vi "XYStage.GetProtectedEventsRegistration.vi"(8 "error in (no error)":errorcluster, 11 "XYStage in":refnum<class "XYStage.lvclass">) -> (0 "error out":errorcluster, 2 "XYStage Protected Events":refnum<event-registration>, 3 "XYStage out":refnum<class "XYStage.lvclass">)   [LabVIEW 2017, in "XYStage.lvclass"]
uses:
  XYStage.lvclass
  Typedefs/ProtectedEvents--Cluster.ctl
  Typedefs/ProtectedEvents--XYStage.StatusUpdated.ctl
  Typedefs/XYStage.Axis--Enum.ctl
  Typedefs/XYStage.DeviceStatus--Enum.ctl
  Typedefs/ProtectedEvents--XYStage.MoveResultReported.ctl
  Typedefs/Coordinates--Cluster.ctl
  Typedefs/Coordinates.Units--Cluster.ctl
  Typedefs/Coordinates.Counts--Cluster.ctl
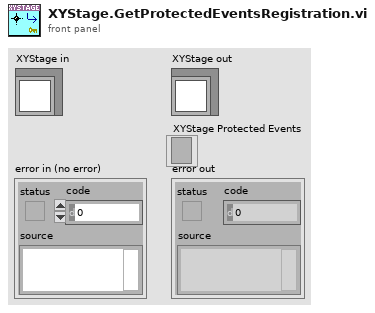
[diagram p1: front panel]
types:
  T1 = typedef "XYStage.lvclass/ProtectedEvents--Cluster.ctl" = cluster{"StatusUpdated":refnum<user-event>, "MoveResultReported":refnum<user-event>}
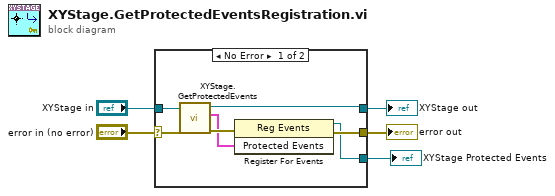
[diagram p0: block diagram]
diagram:
  n1 = case shown="No Error" "error in (no error)" {
    selector: "error in (no error)" -> [w9 w14]
    tunnel: [w12 w14] -> w4
    tunnel: [w7 w13] -> w2
    tunnel: "XYStage in" -> [w10 w13]
    tunnel: [w11 _] -> w1
    frame No Error {
      n2 = call "XYStage.GetProtectedEvents.vi"("error in (no error)"=w9, "XYStage"=w10) -> ("error out"=w8:errorcluster, "Protected Events"=w6:T1, "XYStage out"=w7:refnum<class "XYStage.lvclass">)  [unwired: 7 in]
      n3 = register-events(error in=w8, w6) -> (reference out=w11:refnum<event-registration>, error out=w12:errorcluster)  [unwired: 1 in]
    }
    frame Error {
    }
  }
  "error out" <- w4
  "XYStage out" <- w2
  "XYStage Protected Events" <- w1
